vi "Main.vi"() -> ()   [LabVIEW 2015]
doc: "This template is for the Queued Message Handler design pattern.\n\nThe Event Handling Loop generates messages based on user interface actions.\n\nThe Message Handling Loop processes messages generated by the Event Handling Loop, or by other messages. The messages are string values, so new messages can be added easily to the Message Cases case structure in the Message Handling Loop. Each message cluster can also provide an optional value for Message Data, which is a variant that can be converted to whatever message-specific data is required."
uses:
  support/Type Definitions/UI Data.ctl
  support/Status Logger/Status Log.ctl
  Report/TypeDefs/Report state.ctl
  TCP/TypeDefs/TCP Data.ctl
  <vilib>/Utility/error.llb/DialogType.ctl
  DAQ/TypeDefs/DAQ data.ctl
  support/Global names.vi
  support/Message Queue/Enqueue Message (Single).vi
  <vilib>/Utility/error.llb/Error Cluster From Error Code.vi
  <vilib>/ErrorRing/Error Ring.xnode
  support/Message Queue/Message Queue.lvlib
  support/User Event - EHL Stop/User Event - EHL Stop.lvlib
  Model/Model.lvlib
  DAQ/DAQ.lvlib
  PLC/PLC.lvlib
  Logger/Logger.lvlib
  TCP/TCP.lvlib
  Report/Report.lvlib
panel:
  out "Power status":bool
  in  "Remote":bool
  in  "Abort":bool
  in  "Stop Line":bool
  in  "Start Line":bool
  out "Status":string
  in  "Tab Control":T1(tab)
  in  "Power switch":bool
  in  "Positon":dbl(slide) scale=0.0..20.0
  in  "Dispose":bool
  in  "Pump":bool
  in  "Flow [l/s]":dbl=10.0
  in  "Potentiometer (AI)":tag
  in  "LED (DO)":tag
  in  "Bistable switch (DI)":tag
  in  "Monostable switch (DI)":tag
  in  "Send":bool
  in  "Message to send":string
  out "Message received":string
  in  "Disconnect":bool
  in  "Connect":bool
  out "Connected?":bool
  in  "Type":enum16{"Server", "Client"}(ring)
  in  "Port":u16
  in  "IP":string
  out "Current machine IP":string
  in  "Current printer":u16(ring) items=["Wyœlij do programu OneNote 2013", "OneNote", "Microsoft XPS Document Writer", "Microsoft Print to PDF", "Fax"]
  in  "Check printers":bool
  in  "Print report":bool
  in  "TDMS View":bool
  in  "Exit":bool
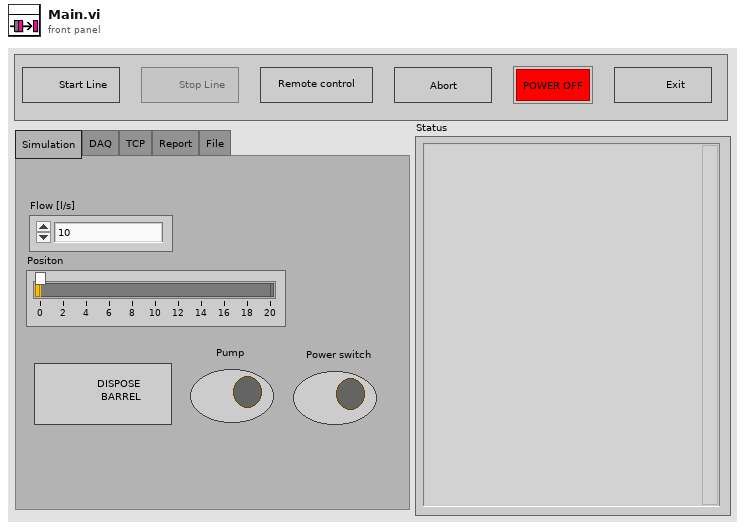
[diagram p1: front panel]
types:
  T1 = enum32{"Simulation", "DAQ", "TCP", "Report", "File"}
  T2 = typedef "Status Log.ctl" = enum16{"Close file", "Open Status file", "Add Status", "Show Status File"}
  T3 = typedef "UI Data.ctl" = cluster{"Start Line Ref":refnum<vi>, "Stop Line Ref":refnum<vi>, "Data Display Ref":refnum<vi>, "Exit Button Ref":refnum<vi>, "Pump Ref":refnum<vi>, "Dispose Ref":refnum<vi>, "Flow Ref":refnum<vi>, "Position Ref":refnum<vi>, "Tab Ref":refnum<vi>, "Print report":refnum<vi>, "Remote":refnum<vi>, "Connection status":refnum<vi>, "Abort":refnum<vi>, "Power status":refnum<vi>, "Power switch":refnum<vi>}
  T4 = typedef "Notifiers.lvlib/Notifiers.ctl" = cluster{"PLC":refnum<notifier>, "Model":refnum<notifier>, "DAQ":refnum<notifier>, "Log":refnum<notifier>, "TCP":refnum<notifier>}
  T5 = typedef "Message Queue.lvlib/All Message Queues.ctl" = cluster{"UI":refnum<queue>, "Model":refnum<queue>, "DAQ":refnum<queue>, "PLC":refnum<queue>, "Log":refnum<queue>, "TCP":refnum<queue>}
  T6 = typedef "Report.lvlib/Report state.ctl" = enum16{"Create report", "Save data", "Save report", "Available printers", "Print report", "Close report", "Reset State"}
  T7 = typedef "TCP.lvlib/TCP Data.ctl" = cluster{"Type":enum16{"Server", "Client"}, "IP":string, "Port":u16, "connection ID":refnum<k5>, "Connected?":bool, "Data":string}
  T8 = typedef "DialogType.ctl" = u16
  T9 = typedef "DAQ.lvlib/DAQ data.ctl" = cluster{"Power switch (DI)":cluster{"Channel":tag, "Data":bool}, "Dispose barrel (DI)":cluster{"Channel":tag, "Data":bool}, "Pump status (DO)":cluster{"Channel":tag, "Data":bool}, "Barrel position (AI)":cluster{"Channel":tag, "Data":dbl}}
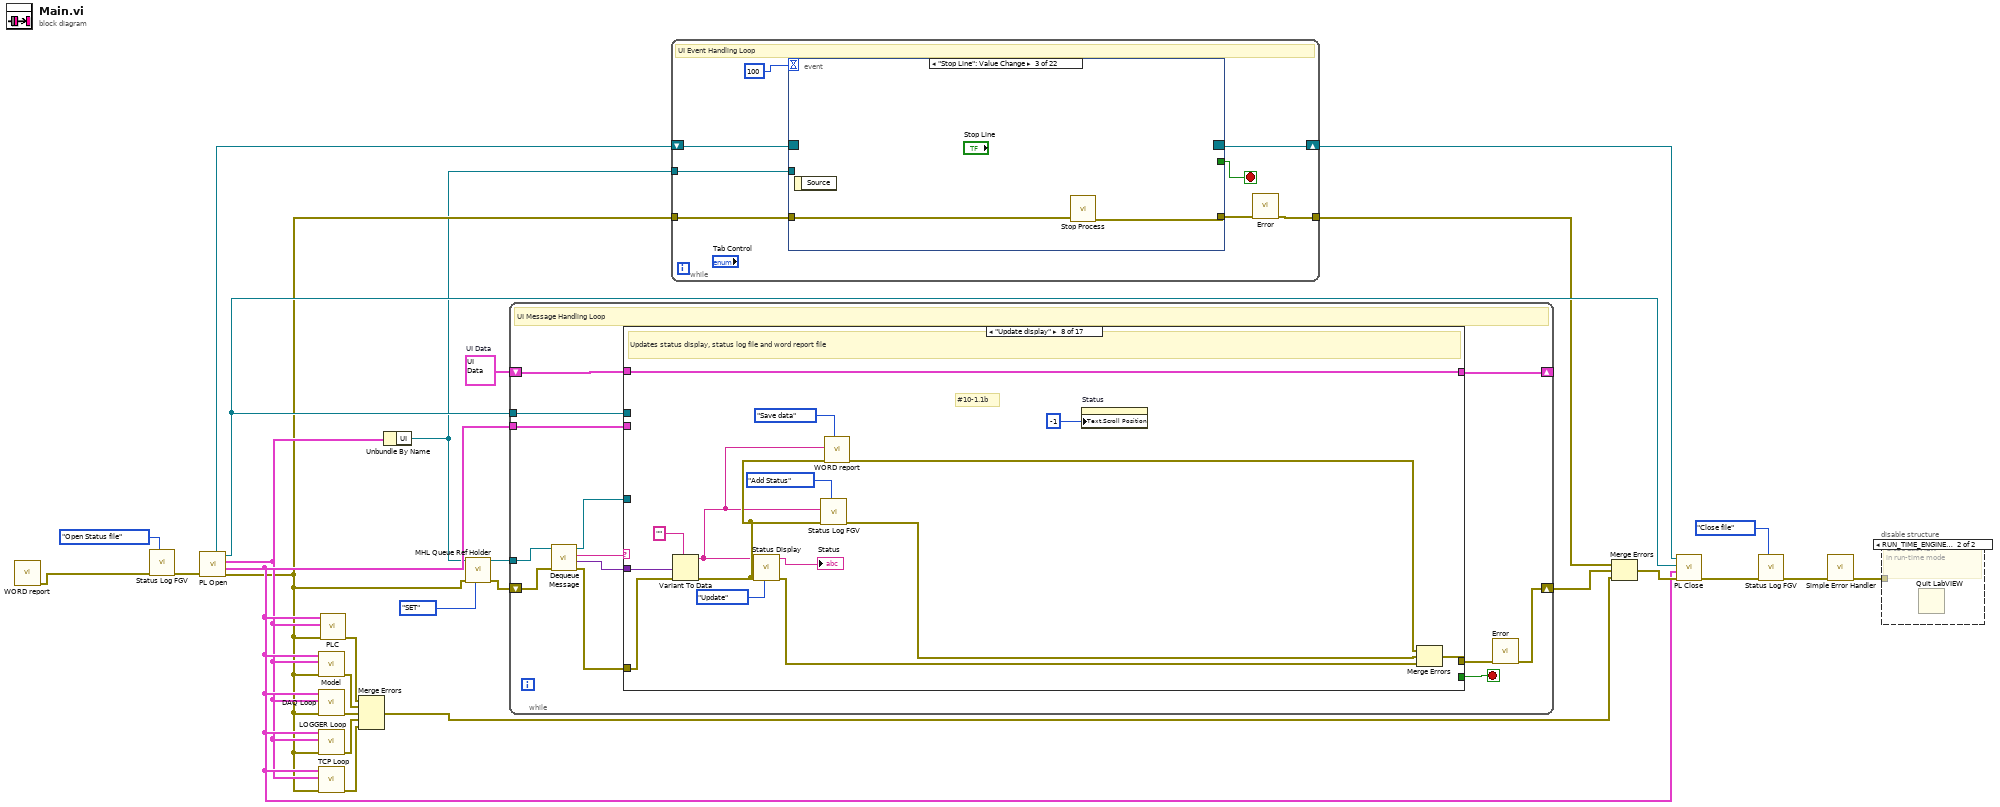
[diagram p0: block diagram]
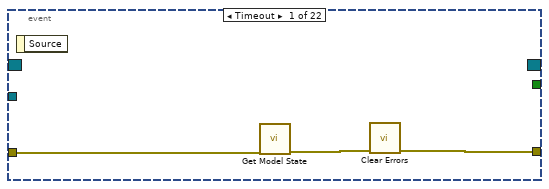
[diagram p2: hidden frame]
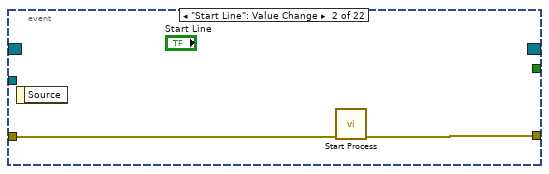
[diagram p3: hidden frame]
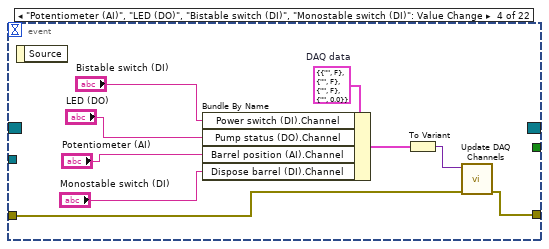
[diagram p4: hidden frame]
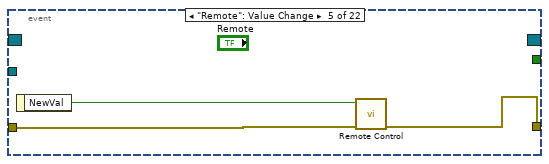
[diagram p5: hidden frame]
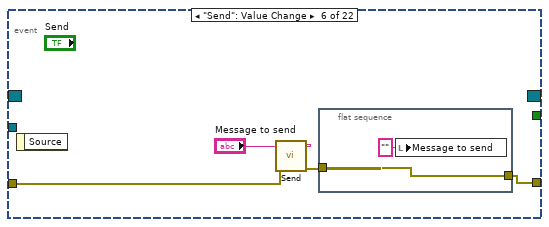
[diagram p6: hidden frame]
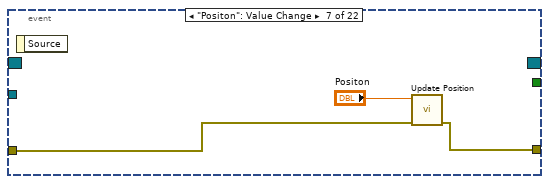
[diagram p7: hidden frame]
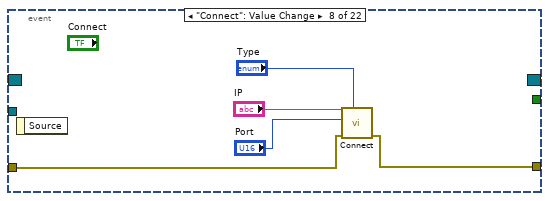
[diagram p8: hidden frame]
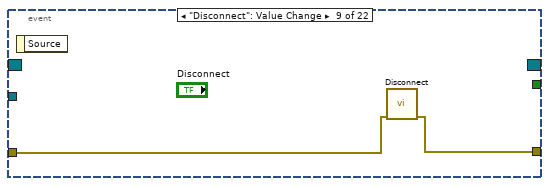
[diagram p9: hidden frame]
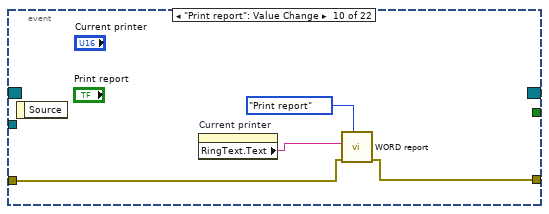
[diagram p10: hidden frame]
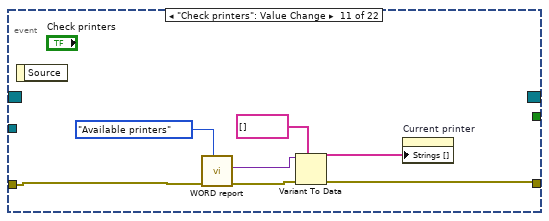
[diagram p11: hidden frame]
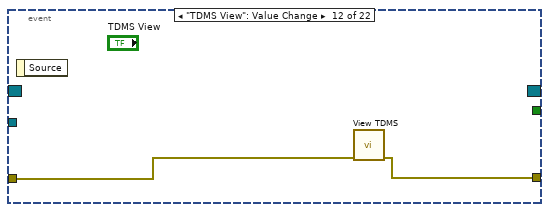
[diagram p12: hidden frame]
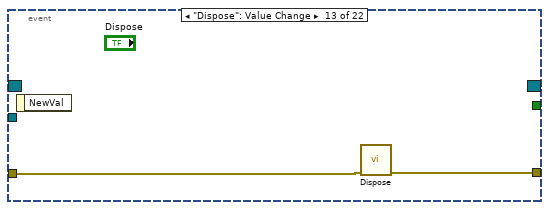
[diagram p13: hidden frame]
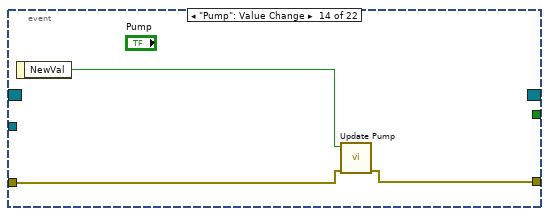
[diagram p14: hidden frame]
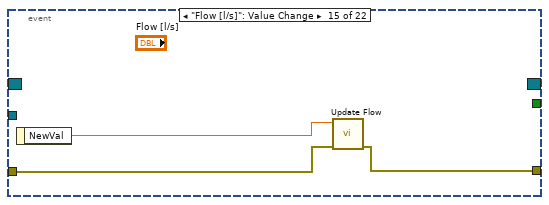
[diagram p15: hidden frame]
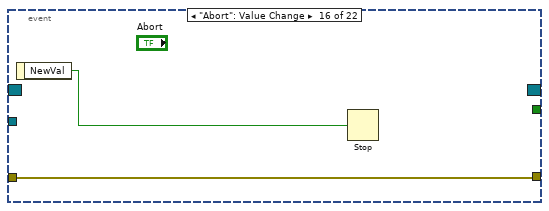
[diagram p16: hidden frame]
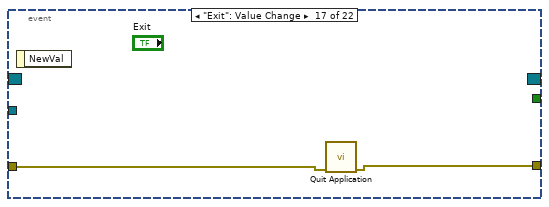
[diagram p17: hidden frame]
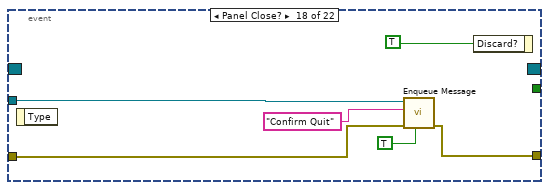
[diagram p18: hidden frame]
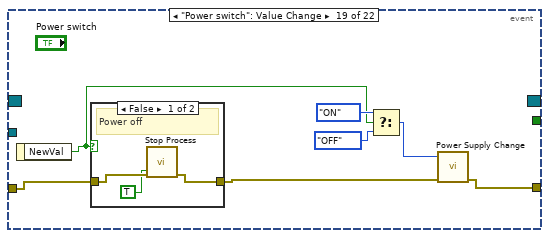
[diagram p19: hidden frame]
diagram:
  w26 = T3 {"Start Line Ref"=refnum, "Stop Line Ref"=refnum, "Data Display Ref"=refnum, "Exit Button Ref"=refnum, "Pump Ref"=refnum, "Dispose Ref"=refnum, "Flow Ref"=refnum, "Position Ref"=refnum, "Tab Ref"=refnum, "Print report"=refnum, "Remote"=refnum, "Connection status"=refnum, "Abort"=refnum, "Power status"=refnum, "Power switch"=refnum}  # UI Data
  n1 = call "WORD report.vi"() -> ("error out"=w1:errorcluster)  [unwired: 10 in, 1 out]
  n2 = call "Status Log FGV.vi"("Action"=Status_Log."Open Status file", "error in"=w1) -> ("error out"=w21:errorcluster)  [unwired: 9 in]
  n3 = call "PL Open.vi"("error in"=w21) -> ("error out"=w5:errorcluster, "Notifiers"=w14:T4, "Queues"=w13:T5, "User Event"=w24:refnum<user-event>, "Event Registration Refnum"=w16:refnum<event-registration>)  [unwired: 6 in]
  n4 = call "Model.vi"("error in"=w5, "Queues"=w13, "Notifiers"=w14) -> ("error out"=w11:errorcluster)  [unwired: 8 in]
  n5 = call "DAQ Loop.vi"("error in"=w5, "Queues"=w13, "Notifiers"=w14) -> ("error out"=w10:errorcluster)  [unwired: 8 in]
  n6 = call "LOGGER Loop.vi"("error in"=w5, "Queues"=w13, "Notifiers"=w14) -> ("error out"=w9:errorcluster)  [unwired: 8 in]
  n7 = call "TCP Loop.vi"("error in"=w5, "Queues"=w13, "Notifiers"=w14) -> ("error out"=w8:errorcluster)  [unwired: 8 in]
  n8 = call "PLC.vi"("error in"=w5, "Message Queues"=w13, "Notifiers"=w14) -> ("error out"=w12:errorcluster)  [unwired: 8 in]
  n9 = Merge Errors(w12, w11, w10, w9, w8) -> (w7:errorcluster)
  n10 = Unbundle By Name(w13) -> ("UI"=w2:refnum<queue>)
  n11 = call "MHL Queue Ref Holder.vi"("Action"=enum16{"GET", "SET"}."SET", "error in"=w5, "Message Queue In"=w2) -> ("error out"=w4:errorcluster, "Input Message Queue"=w6:refnum<queue>)  [unwired: 7 in]
  n12 = while {
    shift-right: [w39] -> _
    shift-left: w26 -> [w40]
    tunnel: w24 -> [w37]
    tunnel: w14 -> [w33]
    shift-right: [w29] -> w20
    shift-left: w4 -> [w36]
    tunnel: w6 -> [w31]
    stop <- w38 stop-if-true
    # "UI Message Handling Loop"
    n13 = call "Dequeue Message.vi"("error in (no error)"=w36, "Message Queue"=w31) -> ("error out"=w35:errorcluster, "Message Data"=w32:variant, "Message"=w28:string, "dup Message Queue"=w34:refnum<queue>)  [unwired: 6 in]
    n14 = case "Message Cases" shown="\"Update display\"" w28 {
      selector: w28 -> [_ _ _ _ _ _ _ _ _ _ _ _ _ _ _ _ w286]
      tunnel: w34 -> [w42 _ _ _ _ _ _ _ _ _ _ _ w232 w238 w274 _ _]
      tunnel: w35 -> [w43 w49 w72 w107 w111 w143 w161 w166 w181 w193 w221 w224 w233 w240 w257 w281 _]
      tunnel: [w41 w49 w82 w108 w125 w145 w157 w167 w182 w187 w217 w223 w230 w237 w261 w275 w285] -> w30
      tunnel: w40 -> [w44 w63 w93 w109 w130 w155 w156 w172 w185 w186 w199 w228 w234 w244 w266 w280 w287]
      tunnel: [w44 w50 w93 w109 w130 w155 w156 w172 w185 w186 w199 w228 w234 w244 w266 w280 w287] -> w39
      tunnel: [_ _ _ _ _ _ _ _ _ _ _ _ _ _ TRUE _ _] -> w38
      tunnel: w32 -> [_ _ _ _ _ _ w160 w176 w179 w192 w220 w227 _ _ w268 _ _]
      tunnel: w37 -> [_ _ _ _ _ _ _ _ _ _ _ _ _ _ w271 _ _]
      tunnel: w33 -> [_ _ _ _ _ _ _ _ _ _ _ _ _ w243 _ _ _]
      frame "Initialize" {
        w45 = string[] ["Initialize references", "Initialize controls", "Initialize PLC"]  # Message
        # "Prepare application initialization procedure"
        n15 = call "Enqueue Message (Array).vi"("error in (no error)"=w43, "Message Array"=w45, "Message Queue"=w42) -> ("error out"=w41:errorcluster)  [unwired: 7 in, 1 out]
      }
      frame "Initialize references" {
        # "Link references to UI objects"
        n16 = control-ref of="Power switch"() -> (w46:refnum<vi>)
        n17 = control-ref of="Stop Line"() -> (w60:refnum<vi>)
        n18 = control-ref of="Flow [l/s]"() -> (w57:refnum<vi>)
        n19 = control-ref of="Dispose"() -> (w58:refnum<vi>)
        n20 = control-ref of="Exit"() -> (w62:refnum<vi>)
        n21 = control-ref of="Start Line"() -> (w61:refnum<vi>)
        n22 = control-ref of="Pump"() -> (w59:refnum<vi>)
        n23 = Bundle By Name(cluster=w63, "Exit Button Ref"=w62, "Start Line Ref"=w61, "Stop Line Ref"=w60, "Pump Ref"=w59, "Dispose Ref"=w58, "Flow Ref"=w57, "Power switch"=w46) -> (w56:T3)
        n24 = control-ref of="Tab Control"() -> (w54:refnum<vi>)
        n25 = control-ref of="Remote"() -> (w52:refnum<vi>)
        n26 = control-ref of="Connection status"() -> (w51:refnum<vi>)
        n27 = control-ref of="Positon"() -> (w55:refnum<vi>)
        n28 = control-ref of="Print report"() -> (w53:refnum<vi>)
        n29 = control-ref of="Power status"() -> (w47:refnum<vi>)
        n30 = control-ref of="Abort"() -> (w48:refnum<vi>)
        n31 = Bundle By Name(cluster=w56, "Position Ref"=w55, "Tab Ref"=w54, "Print report"=w53, "Remote"=w52, "Connection status"=w51, "Abort"=w48, "Power status"=w47) -> (w50:T3)
      }
      frame "Initialize controls" {
        w81 = "" ("Data received")
        w64 = TRUE ("Enabled")
        w65 = FALSE ("Enabled")
        # "Initialize activity and values of UI objects"
        n32 = Unbundle By Name(w93) -> ("Stop Line Ref"=w106:refnum<vi>, "Print report"=w88:refnum<vi>)
        n33 = Current VI's Menubar() -> (w67:refnum<k9>)
        n34 = Build Array(w106, w88) -> (w105:refnum<vi>[])
        n35 = call "Enable Multiple Controls.vi"("error in"=w72, "Enabled"=w65, "References"=w105) -> ("error out"=w102:errorcluster)  [unwired: 8 in]
        n36 = Set Menu Item Info(7:"Stop" ("item tag"), 8:w72, 9:w65, 11:w67) -> (0:w70:errorcluster, 3:w66:refnum<k9>)  [unwired: 3 in]
        n37 = Unbundle By Name(w93) -> ("Exit Button Ref"=w104:refnum<vi>, "Start Line Ref"=w103:refnum<vi>)
        n38 = call "Power Supply Change.vi"("error in"=w72, "Power status"=enum16{"OFF", "ON"}."OFF") -> ("error out"=w78:errorcluster)  [unwired: 9 in]
        n39 = Build Array(w104, w103) -> (w101:refnum<vi>[])
        n40 = call "Enable Multiple Controls.vi"("error in"=w102, "Enabled"=w64, "References"=w101) -> ("error out"=w96:errorcluster)  [unwired: 8 in]
        n41 = Set Menu Item Info(7:"Start" ("item tag"), 8:w70, 9:w64, 11:w66) -> (0:w68:errorcluster)  [unwired: 3 in, 1 out]
        n42 = Unbundle By Name(w93) -> ("Exit Button Ref"=w100:refnum<vi>, "Start Line Ref"=w99:refnum<vi>, "Stop Line Ref"=w98:refnum<vi>, "Pump Ref"=w97:refnum<vi>, "Remote"=w87:refnum<vi>, "Connection status"=w86:refnum<vi>, "Abort"=w85:refnum<vi>, "Power status"=w84:refnum<vi>, "Power switch"=w74:refnum<vi>)
        n43 = call "Status Display.vi"("Action"=enum16{"Update", "Clear"}."Clear", "error in"=w78) -> ("error out"=w77:errorcluster, "Status"=w75:string)  [unwired: 8 in]
        n44 = local write "Status"(w75) -> ()
        n45 = Build Array(w100, w99, w98, w97, w87, w86, w85, w84, w74) -> (w94:refnum<vi>[])
        n46 = call "Value Multiple Boolean Controls.vi"("error in"=w96, "Value"=FALSE ("Enabled"), "References"=w94) -> ("error out"=w92:errorcluster)  [unwired: 8 in]
        n47 = Unbundle By Name(w93) -> ("Position Ref"=w91:refnum<vi>)
        n48 = Build Array(w91) -> (w90:refnum<vi>[])
        n49 = call "Value Multiple Numeric Controls.vi"("error in"=w92, "Value"=0.0, "References"=w90) -> ("error out"=w80:errorcluster)  [unwired: 8 in]
        n50 = local write "Message received"(w81) -> ()
        n51 = local write "Message to send"(w81) -> ()
        n52 = call "Update Display.vi"("error in"=w80, "Message string"="UI initialized") -> ("error out"=w69:errorcluster)  [unwired: 9 in]
        n53 = Merge Errors(w69, w68, w77) -> (w82:errorcluster)
      }
      frame "Initialize PLC" {
        # "Initialize Production Line Controller"
        n54 = call "Initialize.vi"("error in"=w107) -> ("error out"=w108:errorcluster)  [unwired: 10 in]
      }
      frame "Start process" {
        w117 = TRUE ("Enabled")
        w121 = FALSE ("Enabled")
        # "#10-1.1a"
        # "Starts process: start PLC, open logger file, create reports files, enable/disable UI controls and update status display"
        n55 = Unbundle By Name(w130) -> ("Exit Button Ref"=w114:refnum<vi>, "Start Line Ref"=w126:refnum<vi>, "Stop Line Ref"=w129:refnum<vi>)
        n56 = Build Array(w114, w126) -> (w131:refnum<vi>[])
        n57 = Build Array(w129) -> (w128:refnum<vi>[])
        n58 = call "WORD report.vi"("Action"=Report_state."Create report", "error in"=w111) -> ("error out"=w110:errorcluster)  [unwired: 8 in, 1 out]
        n59 = call "Start.vi"("error in"=w111) -> ("error out"=w127:errorcluster)  [unwired: 10 in]
        n60 = call "Enable Multiple Controls.vi"("error in"=w111, "Enabled"=w117, "References"=w128) -> ("error out"=w119:errorcluster)  [unwired: 8 in]
        n61 = call "Enable Multiple Controls.vi"("error in"=w111, "Enabled"=w121, "References"=w131) -> ("error out"=w123:errorcluster)  [unwired: 8 in]
        n62 = global read "Global names.vi" "Starting"() -> (w115:string)
        n63 = Current VI's Menubar() -> (w116:refnum<k9>)
        n64 = call "Update Display.vi"("error in"=w127, "Message string"=w115) -> ("error out"=w113:errorcluster)  [unwired: 9 in]
        n65 = Set Menu Item Info(7:"Start" ("item tag"), 8:w123, 9:w121, 11:w116) -> (0:w122:errorcluster)  [unwired: 3 in, 1 out]
        n66 = Set Menu Item Info(7:"Stop" ("item tag"), 8:w119, 9:w117, 11:w116) -> (0:w118:errorcluster)  [unwired: 3 in, 1 out]
        n67 = Merge Errors(w113, w110, w122, w118) -> (w125:errorcluster)
      }
      frame "Stop process" {
        w134 = FALSE ("Enabled")
        w135 = TRUE ("Enabled")
        # "Stops process: stop PLC, close logger file, save and close report files, enable/disable UI controls and update status display"
        n68 = Unbundle By Name(w155) -> ("Exit Button Ref"=w132:refnum<vi>, "Start Line Ref"=w148:refnum<vi>, "Stop Line Ref"=w154:refnum<vi>)
        n69 = call "Stop.vi"("error in"=w143) -> ("error out"=w150:errorcluster)  [unwired: 10 in]
        n70 = Build Array(w154) -> (w144:refnum<vi>[])
        n71 = Build Array(w132, w148) -> (w152:refnum<vi>[])
        n72 = global read "Global names.vi" "Stopping"() -> (w133:string)
        n73 = Build Array (concatenate)(w152, w144) -> (w151:refnum<vi>[])
        n74 = call "Enable Multiple Controls.vi"("error in"=w143, "Enabled"=w135, "References"=w152) -> ("error out"=w140:errorcluster)  [unwired: 8 in]
        n75 = call "Enable Multiple Controls.vi"("error in"=w143, "Enabled"=w134, "References"=w144) -> ("error out"=w147:errorcluster)  [unwired: 8 in]
        n76 = call "Value Multiple Boolean Controls.vi"("error in"=w143, "Value"=FALSE, "References"=w151) -> ("error out"=w146:errorcluster)  [unwired: 8 in]
        n77 = call "Update Display.vi"("error in"=w150, "Message string"=w133) -> ("error out"=w149:errorcluster)  [unwired: 9 in]
        n78 = Current VI's Menubar() -> (w141:refnum<k9>)
        n79 = Set Menu Item Info(7:"Start" ("item tag"), 8:w140, 9:w135, 11:w141) -> (0:w138:errorcluster, 3:w136:refnum<k9>)  [unwired: 3 in]
        n80 = Set Menu Item Info(7:"Stop" ("item tag"), 8:w138, 9:w134, 11:w136) -> (0:w137:errorcluster)  [unwired: 3 in, 1 out]
        n81 = Merge Errors(w149, w137, w147, w146) -> (w145:errorcluster)
      }
      frame "Update IP" {
        # "Update IP address of current machine"
        n82 = Variant To Data(error in=w161, type="", Variant=w160) -> (data=→"Current machine IP":string, error out=w157:errorcluster)
      }
      frame "Update display" {
        # "#10-1.1b"
        # "Updates status display, status log file and word report file"
        n83 = Variant To Data(error in=w166, type="", Variant=w176) -> (data=w162:string, error out=w165:errorcluster)
        n84 = call "Status Display.vi"("Action"=enum16{"Update", "Clear"}."Update", "error in"=w165, "Status line"=w162) -> ("error out"=w168:errorcluster, "Status"=→"Status":string)  [unwired: 7 in]
        n85 = call "Status Log FGV.vi"("Action"=Status_Log."Add Status", "error in"=w165, "Status"=w162) -> ("error out"=w169:errorcluster)  [unwired: 8 in]
        n86 = call "WORD report.vi"("Action"=Report_state."Save data", "error in"=w165, "Data in"=w162) -> ("error out"=w163:errorcluster)  [unwired: 7 in, 1 out]
        n87 = property on="Status" class="Str"("Text.Scroll Position"=-1) -> ()  [unwired: 2 in, 2 out]
        n88 = Merge Errors(w163, w169, w168) -> (w167:errorcluster)
      }
      frame "Update position" {
        # "Programmatically update position of the barrel slider"
        n89 = Variant To Data(error in=w181, type=0.0 ("Value"), Variant=w179) -> (data=w177:dbl, error out=w180:errorcluster)
        n90 = Unbundle By Name(w185) -> ("Position Ref"=w184:refnum<vi>)
        n91 = Build Array(w184) -> (w183:refnum<vi>[])
        n92 = call "Value Multiple Numeric Controls.vi"("error in"=w180, "Value"=w177, "References"=w183) -> ("error out"=w182:errorcluster)  [unwired: 8 in]
      }
      frame "Update Connection UI" {
        w191 = T7 {"Type"=enum."Server", "IP"="", "Port"=0, "connection ID"=refnum, "Connected?"=FALSE, "Data"=""}  # TCP Data
        # "Updates TCP conection UI indicators"
        n93 = Variant To Data(error in=w193, type=w191, Variant=w192) -> (data=w190:T7, error out=w187:errorcluster)
        n94 = Unbundle By Name(w190) -> ("Connected?"=→"Connected?":bool, "Data"=→"Message received":string)
      }
      frame "Power status change" {
        # "Update main switch LED and Start/Stop buttons according to power status change (DAQ DI)"
        n95 = Variant To Data(error in=w221, type=TRUE, Variant=w220) -> (data=w200:bool, error out=w204:errorcluster)
        "Power status" <- w200
        n96 = Unbundle By Name(w199) -> ("Position Ref"=w194:refnum<vi>, "Dispose Ref"=w198:refnum<vi>, "Pump Ref"=w197:refnum<vi>)
        n97 = Unbundle By Name(w199) -> ("Start Line Ref"=w196:refnum<vi>, "Stop Line Ref"=w218:refnum<vi>)
        n98 = Build Array(w194, w198, w197, w196) -> (w195:refnum<vi>[])
        n99 = Build Array(w196) -> (w216:refnum<vi>[])
        n100 = Build Array(w218) -> (w213:refnum<vi>[])
        n101 = Build Array (concatenate)(w216, w213) -> (w215:refnum<vi>[])
        n102 = Current VI's Menubar() -> (w207:refnum<k9>)
        n103 = call "Enable Multiple Controls.vi"("error in"=w204, "Enabled"=w200, "References"=w195) -> ("error out"=w211:errorcluster)  [unwired: 8 in]
        n104 = Set Menu Item Info(7:"Start" ("item tag"), 8:w204, 9:w200, 11:w207) -> (0:w205:errorcluster, 3:w201:refnum<k9>)  [unwired: 3 in]
        n105 = call "Value Multiple Boolean Controls.vi"("error in"=w204, "Value"=FALSE, "References"=w215) -> ("error out"=w210:errorcluster)  [unwired: 8 in]
        n106 = call "Enable Multiple Controls.vi"("error in"=w204, "Enabled"=FALSE, "References"=w213) -> ("error out"=w209:errorcluster)  [unwired: 8 in]
        n107 = Set Menu Item Info(7:"Stop" ("item tag"), 8:w205, 9:FALSE ("enabled"), 11:w201) -> (0:w202:errorcluster)  [unwired: 3 in, 1 out]
        n108 = Merge Errors(w211, w210, w209, w202) -> (w217:errorcluster)
      }
      frame "Error" {
        w222 = T8 2 items=["no dialog", "OK message", "continue or stop message", "OK message + warnings", "continue/stop + warnings"] ("type of dialog (OK msg:1)")
        # "Display error dialog box and quit application"
        n109 = Variant To Data(error in=w224, type=errorcluster {"status"=FALSE, "code"=0, "source"=""} ("error constant"), Variant=w227) -> (data=w225:errorcluster, error out=w223:errorcluster)
        n110 = call <vilib>:"Simple Error Handler.vi"("type of dialog (OK msg:1)"=w222, "error in (no error)"=w225) -> ()  [unwired: 3 in, 5 out]
      }
      frame "Exit" {
        # "Start exit procedure: stop PLC, then send Exit message to PLC and go to PLC confirmation loop"
        n111 = Flush Queue(queue=w232, error in (no error)=w233) -> (error out=w229:errorcluster)  [unwired: 2 out]
        n112 = call "Exit PLC.vi"("error in"=w229) -> ("error out"=w231:errorcluster)  [unwired: 10 in]
        n113 = call "Wait on PLC Exit.vi"("error in"=w231) -> ("error out"=w230:errorcluster)  [unwired: 10 in]
      }
      frame "Wait on PLC exit" {
        # "Wait until PLC shutdown"
        n114 = Unbundle By Name(w243) -> ("PLC"=w242:refnum<notifier>)
        n115 = Wait on Notification(notifier=w242, timeout in ms (-1)=10, error in (no error)=w240) -> (notification=w236:string, timed out?=w239:bool, error out=w235:errorcluster)  [unwired: 1 in, 1 out]
        n116 = case shown="True" w239 {
          tunnel: [w245 w254] -> w237
          tunnel: w235 -> [w246 w251]
          tunnel: w238 -> [_ w252]
          tunnel: w236 -> [_ w247]
          frame True {
            # "Shutdown notification from PLC not received"
            n117 = call "Wait on PLC Exit.vi"("error in"=w246) -> ("error out"=w245:errorcluster)  [unwired: 10 in]
          }
          frame False {
            # "Shutdown notification from PLC received (handshake)"
            n118 = call "Update Display.vi"("error in"=w251, "Message string"=w247) -> ("error out"=w250:errorcluster)  [unwired: 9 in]
            n119 = call "Update Display.vi"("error in"=w250, "Message string"="Application quits" ("Message")) -> ("error out"=w249:errorcluster)  [unwired: 9 in]
            n120 = call-poly "Enqueue Message.vi"("error in (no error)"=w249, "Message"="End program", "Message Queue"=w252) -> ("error out"=w254:errorcluster)  [unwired: 7 in, 1 out]
          }
        }
      }
      frame "End program" {
        # "Shutdown MHL and send exit user event to EHL; reset UI controls"
        n121 = call "Fire User Event - EHL Stop.vi"("error in (no error)"=w257, "User Event - Stop"=w271) -> ("error out"=w256:errorcluster)  [unwired: 9 in]
        n122 = Variant To Data(error in=w257, type=errorcluster {"status"=FALSE, "code"=0, "source"=""} ("error constant"), Variant=w268) -> (data=w269:errorcluster)  [unwired: 1 out]
        n123 = Release Queue(queue=w274, force destroy? (F)=TRUE, error in (no error)=w257) -> (error out=w272:errorcluster)  [unwired: 2 out]
        n124 = call <vilib>:"Simple Error Handler.vi"("error in (no error)"=w269) -> ("error out"=w255:errorcluster)  [unwired: 4 in, 4 out]
        n125 = Merge Errors(w256, w255, w272) -> (w262:errorcluster)
        n126 = Unbundle By Name(w266) -> ("Exit Button Ref"=w265:refnum<vi>, "Abort"=w260:refnum<vi>, "Start Line Ref"=w259:refnum<vi>, "Stop Line Ref"=w258:refnum<vi>)
        n127 = Build Array(w265, w260, w259, w258) -> (w264:refnum<vi>[])
        n128 = call "Value Multiple Boolean Controls.vi"("error in"=w262, "Value"=FALSE, "References"=w264) -> ("error out"=w261:errorcluster)  [unwired: 8 in]
      }
      frame "Confirm Quit" {
        # "Confirm Quit - Message that can confirm whether or not the user wants to exit the application."
        n129 = Two Button Dialog(message="Are you sure?", 1:"Continue" ("F button name (\"Cancel\")"), 2:"Quit" ("T button name (\"OK\")")) -> (T button?=w276:bool)
        n130 = case shown="True" w276 {
          tunnel: w281 -> [w282 w284]
          tunnel: [w282 w283] -> w275
          frame False {
          }
          frame True {
            n131 = call "Quit Application.vi"("error in"=w284) -> ("error out"=w283:errorcluster)  [unwired: 10 in]
          }
        }
      }
      frame Default {
        # "Incorrect message: show error and clear error"
        n132 = xnode "Error Ring"("parameter 0"=w286) -> ("error out"=w285:errorcluster)
      }
    }
    n133 = call "Error.vi"("error in"=w30) -> ("error out"=w29:errorcluster)  [unwired: 10 in]
  }
  n134 = while {
    tunnel: w2 -> [w297]
    shift-right: [w301] -> w27
    shift-left: w16 -> [w302]
    tunnel: [w295] -> w15
    tunnel: w5 -> [w298]
    stop <- w300 stop-if-true
    # "UI Event Handling Loop"
    n135 = event shown="[2] \"Stop Line\": Value Change" {
      selector: w302 -> [_ _ _ _ _ _ _ _ _ _ _ _ _ _ _ _ _ _ _ _ _ _]
      dyn-events: [_ _ _ _ _ _ _ _ _ _ _ _ _ _ _ _ _ _ _ _ _ _] -> w301
      timeout: 100 -> [_ _ _ _ _ _ _ _ _ _ _ _ _ _ _ _ _ _ _ _ _ _]
      tunnel: [_ _ _ _ _ _ _ _ _ _ _ _ _ _ _ _ _ _ _ _ TRUE ("Discard?") _] -> w300
      tunnel: w297 -> [_ _ _ _ _ _ _ _ _ _ _ _ _ _ _ _ _ w368 _ _ _ _]
      tunnel: [w303 w306 w308 w318 w321 w322 w329 w331 w336 w340 w345 w349 w351 w354 w357 w360 w361 w367 w369 w380 w381 w384] -> w296
      tunnel: w298 -> [w305 w307 w309 w317 w320 w323 w328 w332 w337 w341 w348 w350 w352 w355 w358 w360 w362 w363 w371 w380 w381 w383]
      event Timeout {
        n136 = event-data() -> ()  [unwired: 1 in, 1 out]
        n137 = call "Get Model State.vi"("error in (no error)"=w305) -> ("error out"=w304:errorcluster)  [unwired: 10 in]
        n138 = call <vilib>:"Clear Errors.vi"("error in (no error)"=w304) -> ("error out"=w303:errorcluster)  [unwired: 5 in, 1 out]
      }
      event "Start Line": Value Change {
        n139 = event-data() -> ()  [unwired: 1 in, 1 out]
        n140 = call "Start Process.vi"("error in"=w307) -> ("error out"=w306:errorcluster)  [unwired: 10 in]
      }
      event "Stop Line": Value Change {
        n141 = event-data() -> ()  [unwired: 1 in, 1 out]
        n142 = call "Stop Process.vi"("error in"=w309) -> ("error out"=w308:errorcluster)  [unwired: 10 in]
      }
      event "Potentiometer (AI)", "LED (DO)", "Bistable switch (DI)", "Monostable switch (DI)": Value Change {
        w311 = T9 {"Power switch (DI)"={"Channel"="", "Data"=FALSE}, "Dispose barrel (DI)"={"Channel"="", "Data"=FALSE}, "Pump status (DO)"={"Channel"="", "Data"=FALSE}, "Barrel position (AI)"={"Channel"="", "Data"=0.0}}  # DAQ data
        n143 = event-data() -> ()  [unwired: 1 in, 1 out]
        n144 = Bundle By Name(cluster=w311, "Power switch (DI).Channel"="Bistable switch (DI)", "Pump status (DO).Channel"="LED (DO)", "Barrel position (AI).Channel"="Potentiometer (AI)", "Dispose barrel (DI).Channel"="Monostable switch (DI)") -> (w314:T9)
        n145 = To Variant(anything=w314) -> (Variant=w310:variant)
        n146 = call "Update DAQ Channels.vi"("error in"=w317, "Message Data"=w310) -> ("error out"=w318:errorcluster)  [unwired: 9 in]
      }
      event "Remote": Value Change {
        n147 = event-data() -> ("NewVal"=w319:bool)  [unwired: 1 in]
        n148 = call "Remote Control.vi"("error in"=w320, "Remote"=w319) -> ("error out"=w321:errorcluster)  [unwired: 9 in]
      }
      event "Send": Value Change {
        n149 = event-data() -> ()  [unwired: 1 in, 1 out]
        n150 = call "Send.vi"("error in"=w323, "Data"="Message to send") -> ("error out"=w324:errorcluster)  [unwired: 9 in]
        n151 = flat-sequence {
          tunnel: w324 -> [w326]
          tunnel: [w326] -> w322
          frame #0 {
            n152 = local write "Message to send"("" ("Data to send")) -> ()
          }
        }
      }
      event "Positon": Value Change {
        n153 = event-data() -> ()  [unwired: 1 in, 1 out]
        n154 = call "Update Position.vi"("error in (no error)"=w328, "Position"="Positon") -> ("error out"=w329:errorcluster)  [unwired: 9 in]
      }
      event "Connect": Value Change {
        n155 = event-data() -> ()  [unwired: 1 in, 1 out]
        n156 = call "Connect.vi"("Type"="Type", "error in"=w332, "Port"="Port", "IP"="IP") -> ("error out"=w331:errorcluster)  [unwired: 7 in]
      }
      event "Disconnect": Value Change {
        n157 = event-data() -> ()  [unwired: 1 in, 1 out]
        n158 = call "Disconnect.vi"("error in"=w337) -> ("error out"=w336:errorcluster)  [unwired: 10 in]
      }
      event "Print report": Value Change {
        n159 = event-data() -> ()  [unwired: 1 in, 1 out]
        n160 = property on="Current printer" class="Ring (strict)"() -> ("RingText.Text"=w339:string)  [unwired: 2 in, 2 out]
        n161 = call "WORD report.vi"("Action"=Report_state."Print report", "error in"=w341, "Data in"=w339) -> ("error out"=w340:errorcluster)  [unwired: 7 in, 1 out]
      }
      event "Check printers": Value Change {
        n162 = event-data() -> ()  [unwired: 1 in, 1 out]
        n163 = call "WORD report.vi"("Action"=Report_state."Available printers", "error in"=w348) -> ("error out"=w346:errorcluster, "Data out"=w344:variant)  [unwired: 8 in]
        n164 = Variant To Data(error in=w346, type=string[] [], Variant=w344) -> (data=w342:string[], error out=w345:errorcluster)
        n165 = property on="Current printer" class="Ring (strict)"("Strings []"=w342) -> ()  [unwired: 2 in, 2 out]
      }
      event "TDMS View": Value Change {
        n166 = event-data() -> ()  [unwired: 1 in, 1 out]
        n167 = call "View TDMS.vi"("error in"=w350) -> ("error out"=w349:errorcluster)  [unwired: 10 in]
      }
      event "Dispose": Value Change {
        n168 = event-data() -> ()  [unwired: 1 in, 1 out]
        n169 = call "Dispose.vi"("error in (no error)"=w352) -> ("error out"=w351:errorcluster)  [unwired: 10 in]
      }
      event "Pump": Value Change {
        n170 = event-data() -> ("NewVal"=w353:bool)  [unwired: 1 in]
        n171 = call "Update Pump.vi"("error in (no error)"=w355, "Pump State"=w353) -> ("error out"=w354:errorcluster)  [unwired: 9 in]
      }
      event "Flow [l/s]": Value Change {
        n172 = event-data() -> ("NewVal"=w356:dbl)  [unwired: 1 in]
        n173 = call "Update Flow.vi"("error in (no error)"=w358, "Flow"=w356) -> ("error out"=w357:errorcluster)  [unwired: 9 in]
      }
      event "Abort": Value Change {
        n174 = event-data() -> ("NewVal"=w359:bool)  [unwired: 1 in]
        n175 = Stop(stop? (T)=w359) -> ()
      }
      event "Exit": Value Change {
        n176 = event-data() -> ()  [unwired: 1 in, 1 out]
        n177 = call "Quit Application.vi"("error in"=w362) -> ("error out"=w361:errorcluster)  [unwired: 10 in]
      }
      event Panel Close? {
        n178 = event-data() -> ()  [unwired: 1 in, 1 out]
        n179 = call-poly "Enqueue Message.vi"("Priority Message? (F)"=TRUE, "error in (no error)"=w363, "Message"="Confirm Quit", "Message Queue"=w368) -> ("error out"=w367:errorcluster)  [unwired: 6 in, 1 out]
        n180 = event-data("Discard?"=TRUE) -> ()  [unwired: 1 in, 1 out]
      }
      event "Power switch": Value Change {
        n181 = event-data() -> ("NewVal"=w372:bool)  [unwired: 1 in]
        n182 = case shown="False" w372 {
          tunnel: w371 -> [w378 w379]
          tunnel: [w377 w379] -> w370
          frame False {
            # "Power off"
            n183 = call "Stop Process.vi"("Priority Message? (F)"=TRUE, "error in"=w378) -> ("error out"=w377:errorcluster)  [unwired: 9 in]
          }
          frame True {
            # "Power on"
          }
        }
        n184 = Select(t=enum16{"OFF", "ON"}."ON" ("Power status"), s=w372, f=enum16{"OFF", "ON"}."OFF" ("Power status")) -> (s? t:f=w373:enum16{"OFF", "ON"})
        n185 = call "Power Supply Change.vi"("error in"=w370, "Power status"=w373) -> ("error out"=w369:errorcluster)  [unwired: 9 in]
      }
      event Application Instance Close {
        n186 = event-data() -> ()  [unwired: 1 in, 1 out]
      }
      event User Event {
        n187 = event-data() -> ()  [unwired: 1 in, 1 out]
      }
      event Menu Selection (User) {
        n188 = event-data() -> ("ItemTag"=w385:string)  [unwired: 1 in]
        n189 = case shown="\"logdir\"" w385 {
          tunnel: [w386 w389 w390 w394 w395 w397] -> w384
          tunnel: w383 -> [w386 w388 w391 w393 w396 w398]
          frame Default {
          }
          frame "logdir" {
            n190 = global read "Global names.vi" "Status log dir"() -> (w387:string)
            n191 = call "Open Dir.vi"("error in"=w388, "dir"=w387) -> ("error out"=w389:errorcluster)  [unwired: 9 in]
          }
          frame "statuslog" {
            n192 = call "Status Log FGV.vi"("Action"=Status_Log."Show Status File", "error in"=w391) -> ("error out"=w390:errorcluster)  [unwired: 9 in]
          }
          frame "Start" {
            n193 = call "Start Process.vi"("error in"=w393) -> ("error out"=w394:errorcluster)  [unwired: 10 in]
          }
          frame "Stop" {
            n194 = call "Stop Process.vi"("error in"=w396) -> ("error out"=w395:errorcluster)  [unwired: 10 in]
          }
          frame "Exit" {
            n195 = call "Quit Application.vi"("error in"=w398) -> ("error out"=w397:errorcluster)  [unwired: 10 in]
          }
        }
      }
    }
    n196 = call "Error.vi"("error in"=w296) -> ("error out"=w295:errorcluster)  [unwired: 10 in]
  }
  n197 = Merge Errors(w15, w20, w7) -> (w19:errorcluster)
  n198 = call "PL Close.vi"("error in"=w19, "Notifiers"=w14, "User Event"=w24, "Event Registration Refnum in"=w27) -> ("error out"=w25:errorcluster)  [unwired: 7 in]
  n199 = call "Status Log FGV.vi"("Action"=Status_Log."Close file", "error in"=w25) -> ("error out"=w17:errorcluster)  [unwired: 9 in]
  n200 = call <vilib>:"Simple Error Handler.vi"("error in (no error)"=w17) -> ("error out"=w18:errorcluster)  [unwired: 4 in, 4 out]
  n201 = disable-structure shown="RUN_TIME_ENGINE==True" {
    disable-tunnel: w18 -> [_ _]
    frame condition #0 (active) {
    }
    frame condition #1 {
      # "Close LabVIEW\nin run-time mode"
      n202 = Quit LabVIEW() -> ()  [unwired: 1 in]
    }
  }
